vi "cm2nm_update_fiducial_indicator.vi"(1 "Sample Set":T1) -> (0 "Array":u32[](array[numeric]))   [LabVIEW 2011]
uses:
  cm2nm_sample_set.ctl
  cm2nm_coordinate_information_v2.ctl
  Instrument_type_enum_v2.ctl
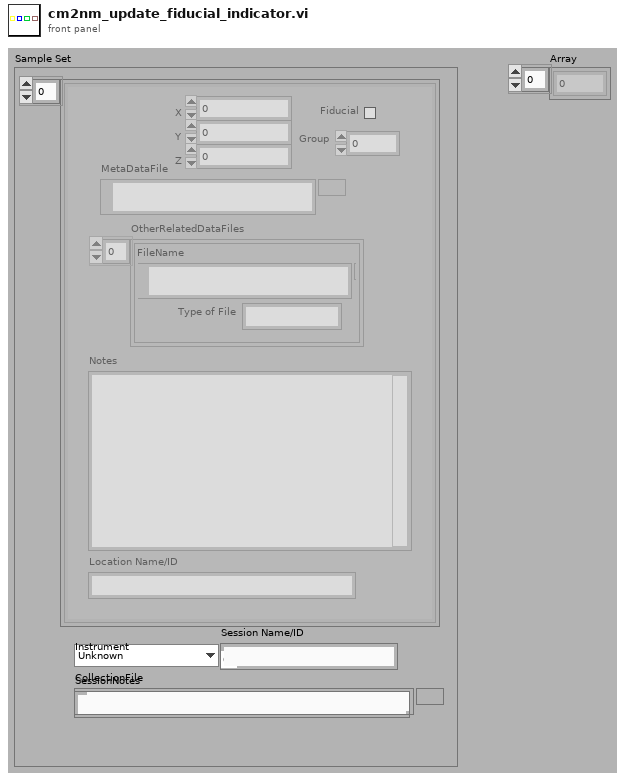
[diagram p1: front panel]
types:
  T1 = typedef "cm2nm_sample_set.ctl" = cluster{"CollectionOfPoints":T2[], "Instrument":T3, "CollectionFile":path, "Session Name/ID":string, "SessionNotes":string}
  T2 = typedef "cm2nm_coordinate_information_v2.ctl" = cluster{"MetaDataFile":path, "X":dbl, "Y":dbl, "Z":dbl, "Group":i32, "Rotation":dbl[unit], "Fiducial":bool, "Magnification":dbl, "Working_Distance":dbl, "Notes":string, "Location Name/ID":string, "OtherRelatedDataFiles":cluster{"Type of File":string, "FileName":path}[], "Available":bool}
  T3 = typedef "Instrument_type_enum_v2.ctl" = enum16{"Unknown", "Philips FEI SEM IRC", "JEOL 7000F EML_MFC", "MXRD MFC", "JEOL_EPMA"}
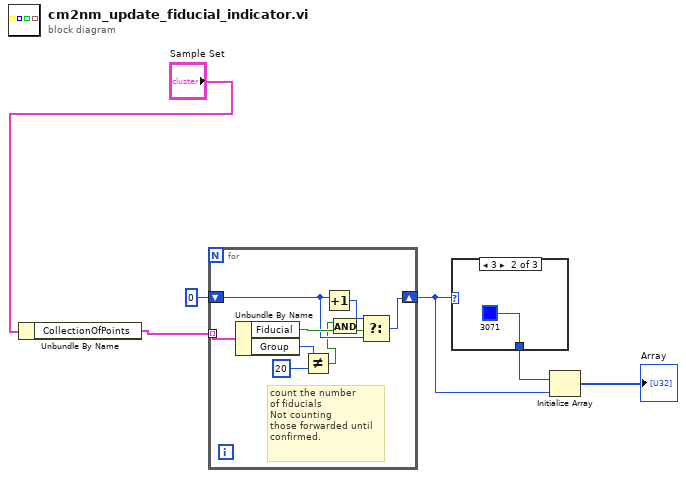
[diagram p0: block diagram]
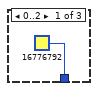
[diagram p2: hidden frame]
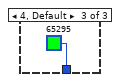
[diagram p3: hidden frame]
diagram:
  n1 = Unbundle By Name("Sample Set") -> ("CollectionOfPoints"=w5:T2[])
  n2 = for {
    tunnel: w5 -> [w15] mode=indexing
    shift-right: [w13] -> w3
    shift-left: 0 -> [w12]
    # "count the number\nof fiducials\nNot counting\nthose forwarded until\nconfirmed."
    n3 = Unbundle By Name(w15) -> ("Fiducial"=w14:bool, "Group"=w10:i32)
    n4 = Not Equal?(x=w10, y=20) -> (x != y?=w7:bool)
    n5 = Increment(x=w12) -> (x+1=w11:i32)
    n6 = And(x=w7, y=w14) -> (x .and. y?=w8:bool)
    n7 = Select(t=w11, s=w8, f=w12) -> (s? t:f=w13:i32)
  }
  n8 = case shown="3" w3 {
    tunnel: [u32 16776792 u32 3071 u32 65295] -> w2
    frame 0..2 {
    }
    frame 3 {
    }
    frame 4, Default {
    }
  }
  n9 = Initialize Array(w2, w3) -> (→"Array":u32[])
